vi "Projeto_SAC.vi"() -> ()   [LabVIEW 2019]
uses:
  <vilib>/Instr/_visa.llb/VISA Configure Serial Port (Instr).vi
panel:
  out "Time":dbl
  in  "Record":bool
  in  "Disturbance to Process":dbl(slide) scale=-10.0..10.0
  in  "?":bool
  out "Process Value out":string
  out "File REF":refnum<file>
  in  "File Path":path
  out "Output Process":string
  out "OP vs t":dbl(graph)
  out "PV vs t":dbl(graph)
  out "Serial Port":refnum<visa-resource-name>
  # "SAC Project - PI CONTROL\n\nJoão Matos\nMaria Loureiro\nMaria Carvalho"
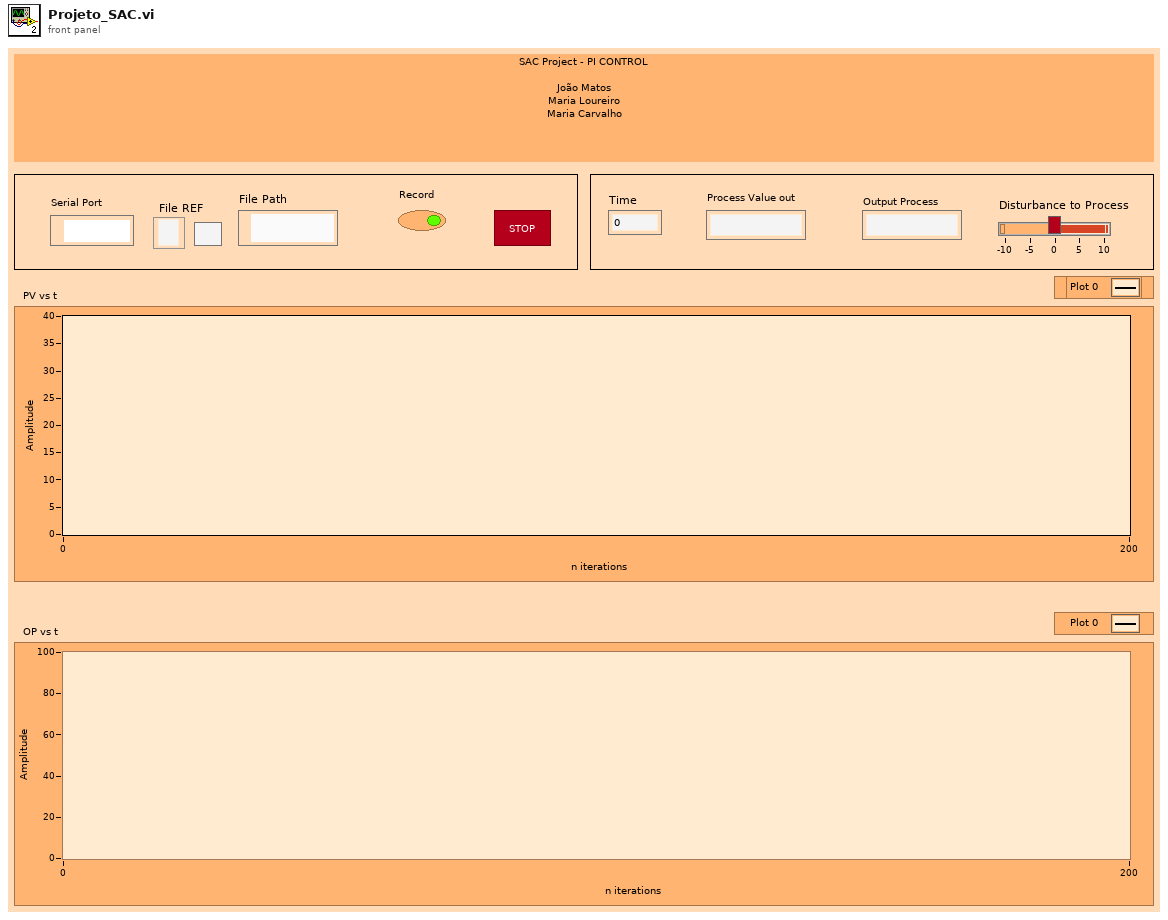
[diagram p1: front panel]
types:
  T1 = enum16{"open", "replace", "create", "open or create", "replace or create", "replace or create with confirmation"}
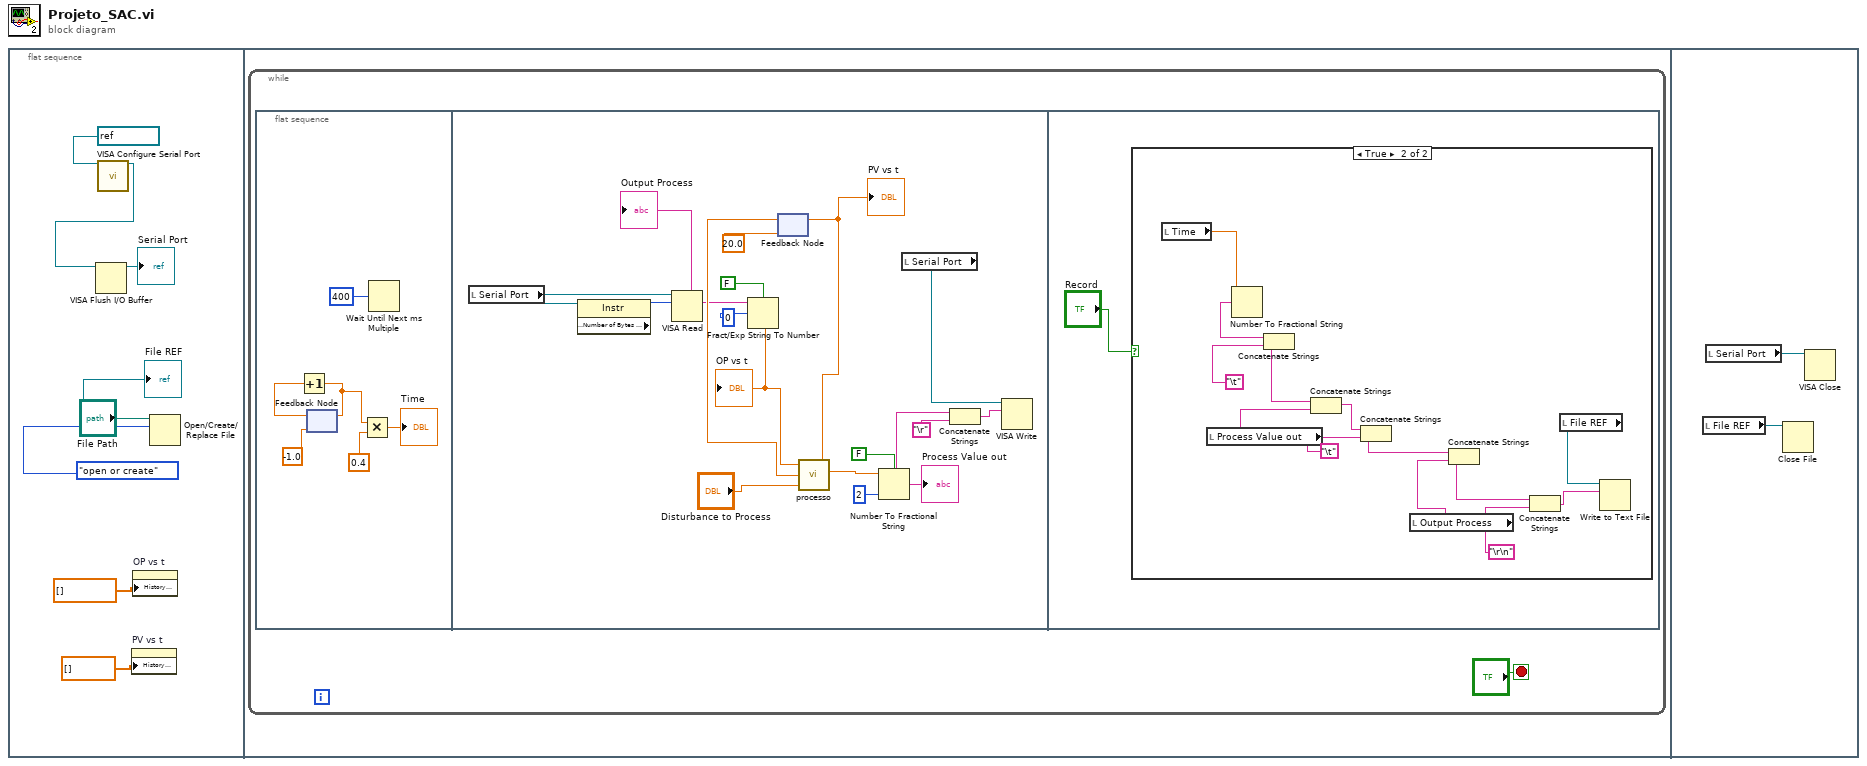
[diagram p0: block diagram]
diagram:
  n1 = flat-sequence {
    frame #0 {
      n2 = call-poly "VISA Configure Serial Port"("VISA resource name"=refnum<visa-resource-name> "COM5") -> ("VISA resource name out"=w7:refnum<visa-resource-name>)  [unwired: 13 in, 1 out]
      n3 = VISA Flush I/O Buffer(VISA resource name=w7) -> (VISA resource name out=→"Serial Port":refnum<visa-resource-name>)  [unwired: 2 in, 1 out]
      n4 = property on="PV vs t" class="WFChart (strict)"("History Data"=dbl[] []) -> ()  [unwired: 2 in, 2 out]
      n5 = property on="OP vs t" class="WFChart (strict)"("History Data"=dbl[] []) -> ()  [unwired: 2 in, 2 out]
      n6 = Open/Create/Replace File(file path (use dialog)="File Path", operation (0:open)=T1."open or create") -> (refnum out=→"File REF":refnum<file>)  [unwired: 4 in, 2 out]
    }
    frame #1 {
      n7 = while {
        stop <- "?" stop-if-true
        n8 = flat-sequence {
          frame #0 {
            n9 = feedback #1(-1.0) -> (w14:dbl)
            n10 = Increment(x=w14) -> (x+1=w12:dbl)
            n11 = feedback-in #1(w12) -> ()
            n12 = Multiply(x=w12, y=0.4) -> (x*y=→"Time":dbl)
            n13 = Wait Until Next ms Multiple(millisecond multiple=u32 400) -> ()  [unwired: 1 out]
          }
          frame #1 {
            n14 = local read "Serial Port"() -> (w26:refnum<visa-resource-name>)
            n15 = property class="Instr"(reference=w26) -> ("Serial Settings:Number of Bytes at Serial Port"=w25:u32)  [unwired: 1 in, 2 out]
            n16 = VISA Read(VISA resource name=w26, byte count=w25) -> (read buffer=w30:string)  [unwired: 1 in, 3 out]
            "Output Process" <- w30
            n17 = Fract/Exp String To Number(use system decimal point (T)=FALSE, string=w30, offset=0) -> (number=w29:dbl)  [unwired: 1 in, 1 out]
            "OP vs t" <- w29
            n18 = feedback #2(20.0 ("PV out")) -> (w31:dbl)
            n19 = call "processo.vi"("DP"="Disturbance to Process", "PV in"=w31, "OP"=w29) -> ("PV out"=w24:dbl)  [unwired: 5 in]
            "PV vs t" <- w24
            n20 = feedback-in #2(w24) -> ()
            n21 = Number To Fractional String(use system decimal point (T)=FALSE, number=w24, precision (6)=i16 2) -> (F-format string=w19:string)  [unwired: 1 in]
            "Process Value out" <- w19
            n22 = local read "Serial Port"() -> (w18:refnum<visa-resource-name>)
            n23 = Concatenate Strings(w19, "\r") -> (w20:string)
            n24 = VISA Write(VISA resource name=w18, write buffer=w20) -> ()  [unwired: 1 in, 3 out]
          }
          frame #2 {
            n25 = case shown="True" "Record" {
              frame False {
              }
              frame True {
                n26 = local read "Time"() -> (w33:dbl)
                n27 = local read "Process Value out"() -> (w34:string)
                n28 = Number To Fractional String(number=w33) -> (F-format string=w43:string)  [unwired: 3 in]
                n29 = Concatenate Strings(w43, "\t") -> (w42:string)
                n30 = Concatenate Strings(w42, w34) -> (w41:string)
                n31 = Concatenate Strings(w41, "\t") -> (w38:string)
                n32 = local read "Output Process"() -> (w39:string)
                n33 = Concatenate Strings(w38, w39) -> (w36:string)
                n34 = Concatenate Strings(w36, "\r\n") -> (w35:string)
                n35 = local read "File REF"() -> (w45:refnum<file>)
                n36 = Write to Text File(file (use dialog)=w45, text=w35) -> ()  [unwired: 2 in, 3 out]
              }
            }
          }
        }
      }
    }
    frame #2 {
      n37 = local read "File REF"() -> (w46:refnum<file>)
      n38 = local read "Serial Port"() -> (w47:refnum<visa-resource-name>)
      n39 = Close File(refnum=w46) -> ()  [unwired: 1 in, 2 out]
      n40 = VISA Close(VISA resource name=w47) -> ()  [unwired: 1 in, 1 out]
    }
  }
